vi "CheckGameBoardContinuityCheck.vi"(8 "error in (no error)":errorcluster, 11 "Board in":T1[][](array[typedef])) -> (0 "error out":errorcluster, 1 "No. of colors":i32, 2 "Pass":bool, 3 "Board out":T1[][](array[typedef]))   [LabVIEW 2020]
uses:
  TypeDef/tiles-key-trunct.ctl
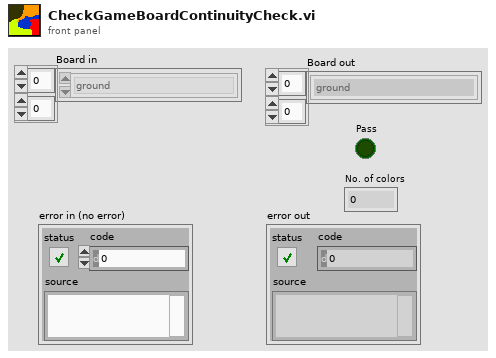
[diagram p1: front panel]
types:
  T1 = typedef "tiles-key-trunct.ctl" = enum16{"ground", "wall", "head (right)", "head (up)", "head (left)", "head (down)", "L-turn (right-up)", "L-turn (up-left)", "L-turn (left-down)", "L-turn (down-right)", "body (right)", "body (up)", "body (left)", "body (down)", "R-turn (right-down)", "R-turn (up-right)", "R-turn (left-up)", "R-turn (down-left)", "tail (right)", "tail (up)", "tail (left)", "tail (down)"}
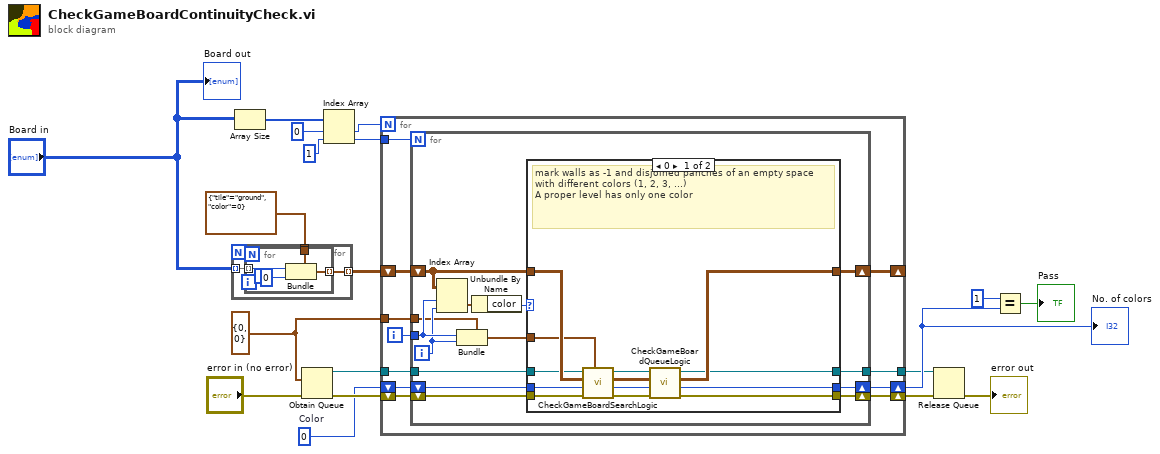
[diagram p0: block diagram]
diagram:
  w8 = 0  # Color
  w12 = cluster{"row":i32, "col":i32} {"row"=0, "col"=0} ("cluster")
  n1 = for {
    tunnel: "Board in" -> [w22] mode=indexing
    tunnel: cluster{"tile":T1, "color":i8} {"tile"=enum."ground", "color"=0} ("cluster") -> [w21]
    tunnel: [w20] -> w11 mode=indexing
    n2 = for {
      tunnel: w22 -> [w26] mode=indexing
      tunnel: w21 -> [w24]
      tunnel: [w23] -> w20 mode=indexing
      n3 = Bundle(cluster=w24, "tile"=w26, "color"=0) -> (w23:cluster{"tile":T1, "color":i8})
    }
  }
  n4 = Array Size(array="Board in") -> (size(s)=w19:i32[])
  n5 = Obtain Queue(element data type=w12, error in (no error)="error in (no error)") -> (queue out=w9:refnum<queue>, error out=w13:errorcluster)  [unwired: 3 in, 1 out]
  n6 = Index Array(array=w19, index #1=0 ("index"), index #2=1 ("index")) -> (element #1=w17:i32, element #2=w18:i32)
  n7 = for {
    N: w17 -> [_]
    shift-right: [w30] -> _
    shift-left: w11 -> [w36]
    tunnel: w12 -> [w35]
    shift-right: [w33] -> w4
    shift-left: w13 -> [w34]
    tunnel: w18 -> [w29]
    shift-right: [w27] -> w6
    shift-left: w8 -> [w28]
    tunnel: w9 -> [w32]
    tunnel: [w31] -> w3
    i -> [w37]
    n8 = for {
      N: w29 -> [_]
      tunnel: w37 -> [w51]
      shift-right: [w42] -> w30
      shift-left: w36 -> [w46]
      tunnel: w35 -> [w49]
      shift-right: [w41] -> w33
      shift-left: w34 -> [w40]
      shift-right: [w38] -> w27
      shift-left: w28 -> [w39]
      tunnel: w32 -> [w44]
      tunnel: [w43] -> w31
      i -> [w50]
      n9 = Index Array(array=w46, index (row)=w51, index (col)=w50) -> (element=w48:cluster{"tile":T1, "color":i8})
      n10 = Bundle(cluster=w49, "row"=w51, "col"=w50) -> (w45:cluster{"row":i32, "col":i32})
      n11 = Unbundle By Name(w48) -> ("color"=w47:i8)
      n12 = case shown="0" w47 {
        tunnel: w46 -> [w64 w67]
        tunnel: w45 -> [w55 _]
        tunnel: w44 -> [w58 w68]
        tunnel: [w59 w68] -> w43
        tunnel: [w60 w67] -> w42
        tunnel: [w56 w66] -> w41
        tunnel: w40 -> [w57 w66]
        tunnel: w39 -> [w54 w65]
        tunnel: [w52 w65] -> w38
        frame 0 {
          # "mark walls as -1 and disjoined pahches of an empty space with different colors (1, 2, 3, ...)\nA proper level has only one color"
          n13 = call "CheckGameBoardSearchLogic.vi"("element"=w55, "error in (no error)"=w57, "Current Color in"=w54, "Coloring Board in"=w64, "Queue in"=w58) -> ("error out"=w61:errorcluster, "Current Color out"=w53:i32, "Coloring Board out"=w63:cluster{"tile":T1, "color":i8}[][], "Queue out"=w62:refnum<queue>)  [unwired: 3 in]
          n14 = call "CheckGameBoardQueueLogic.vi"("error in (no error)"=w61, "Current Color in"=w53, "Coloring Board in"=w63, "Queue in"=w62) -> ("error out"=w56:errorcluster, "Current Color out"=w52:i32, "Coloring Board out"=w60:cluster{"tile":T1, "color":i8}[][], "Queue out"=w59:refnum<queue>)  [unwired: 4 in]
        }
        frame -1, 1, Default {
          # "this element has been visited already - skip"
        }
      }
    }
  }
  "No. of colors" <- w6
  n15 = Release Queue(queue=w3, error in (no error)=w4) -> (error out=→"error out":errorcluster)  [unwired: 1 in, 2 out]
  n16 = Equal?(x=1, y=w6) -> (x = y?=→"Pass":bool)
  "Board out" <- "Board in"
